vi "CC Rd Wr Observation List.vi"(8 "error in (no error)":errorcluster, 9 "filepath":path, 10 "Write? (F:Read)":bool, 11 "Observation List":T1[](array[typedef])) -> (0 "error out":errorcluster, 1 "file":path, 2 "Errors":string[](array[string]), 3 "Observation List":T1[](array[typedef]))   [LabVIEW 2024]
uses:
  typedefs/CC cluster Observation.ctl
  Observation Queue/CC enum Observation Status.ctl
  Telescope/CC cluster Telescope Offsets.ctl
  typedefs/CC cluster Observation Dither Options.ctl
  typedefs/CC enum Dither Selection.ctl
  typedefs/CC cluster RA and DEC.ctl
  <vilib>/Utility/file.llb/Write Delimited Spreadsheet (string).vi
panel:
  out "Header":string[](array[string])
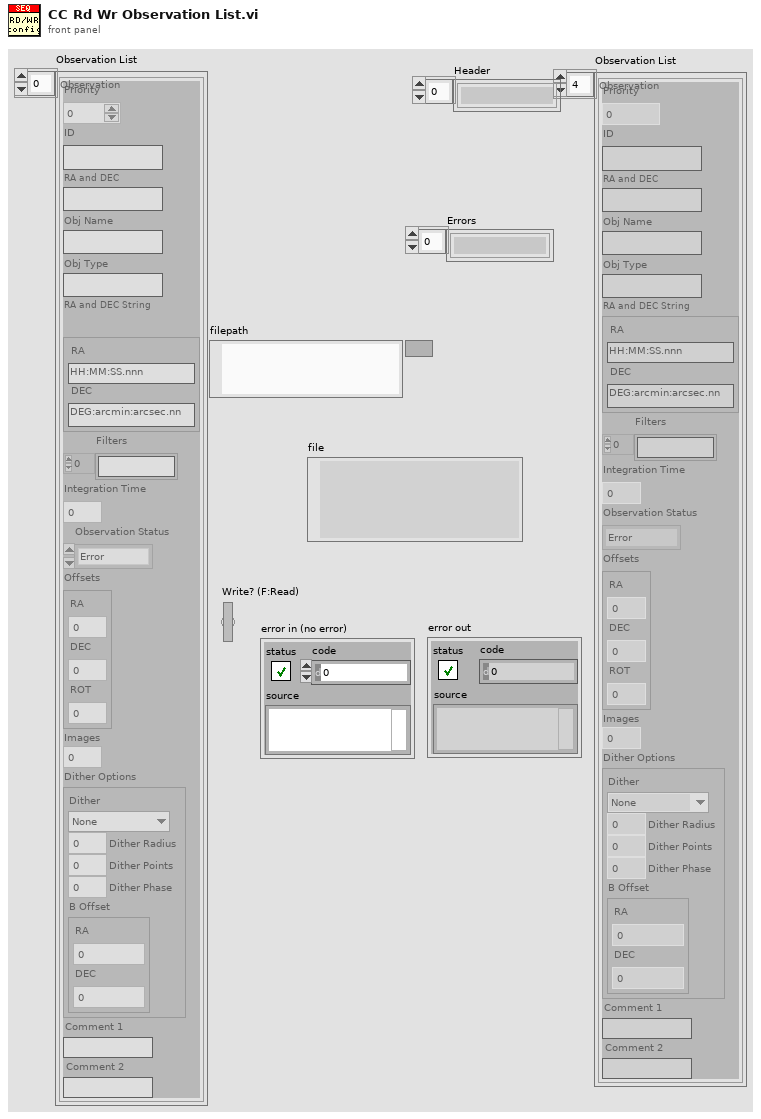
[diagram p1: front panel]
types:
  T1 = typedef "CC cluster Observation.ctl" = cluster{"Priority":i32, "ID":string, "Observer":string, "Obj Name":string, "Obj Type":string, "RA and DEC String":cluster{"RA":string, "DEC":string}, "Filters":string[], "Integration Time":dbl, "Observation Status":T2, "Offsets":T3, "Images":i32, "Dither Options":T4, "Comment 1":string, "Comment 2":string}
  T2 = typedef "CC enum Observation Status.ctl" = enum16{"Ready", "Running", "Done", "Error"}
  T3 = typedef "CC cluster Telescope Offsets.ctl" = cluster{"RA":dbl, "DEC":dbl, "ROT":dbl}
  T4 = typedef "CC cluster Observation Dither Options.ctl" = cluster{"Dither":T5, "Dither Radius":dbl, "Dither Points":i32, "Dither Phase":dbl, "B Offset":T6}
  T5 = typedef "CC enum Dither Selection.ctl" = enum16{"None", "Circle", "Random", "ABBA"}
  T6 = typedef "CC cluster RA and DEC.ctl" = cluster{"RA":dbl, "DEC":dbl}
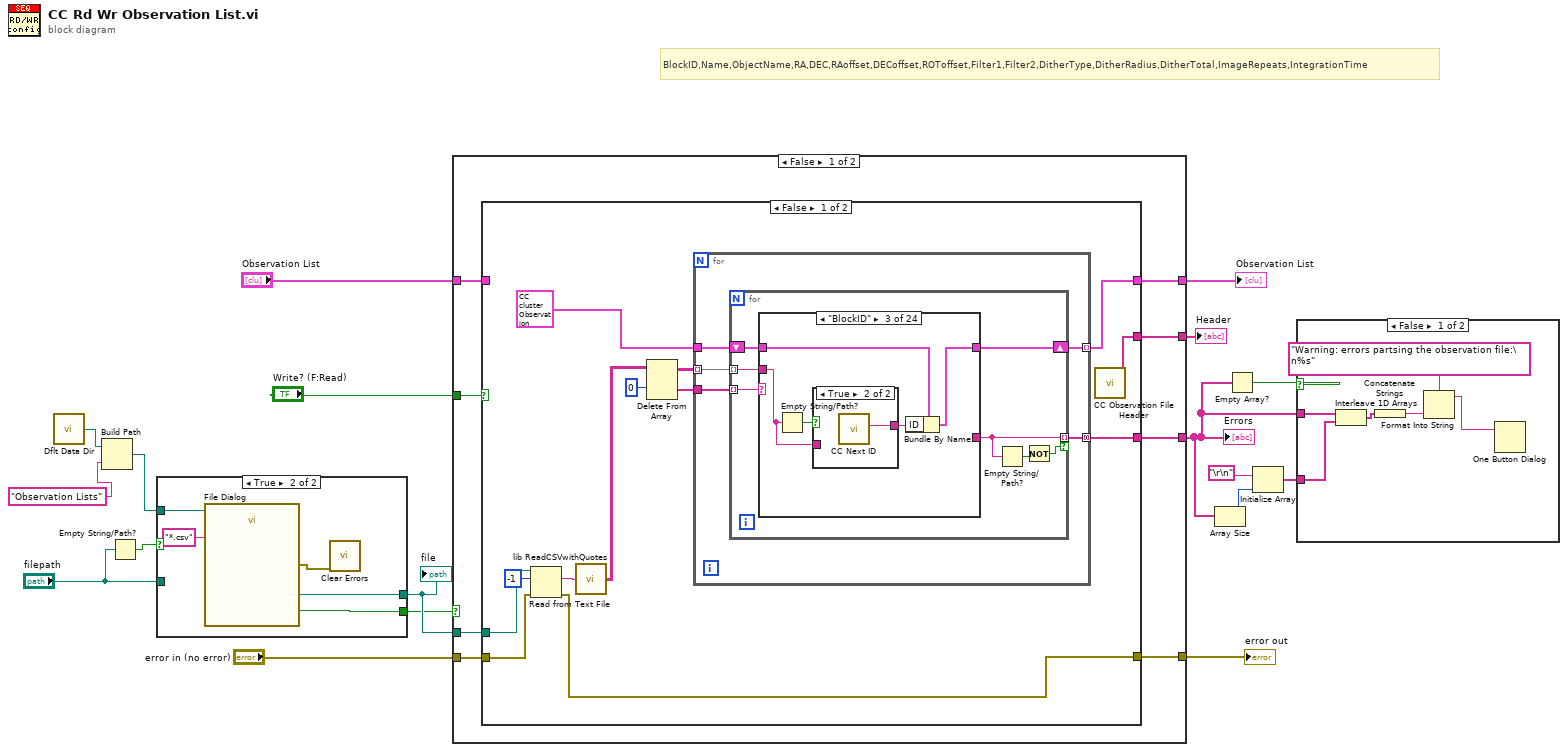
[diagram p0: block diagram]
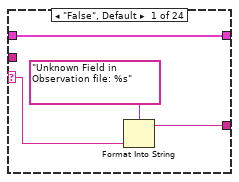
[diagram p3: hidden frame]
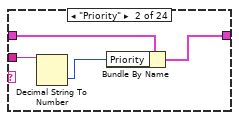
[diagram p4: hidden frame]
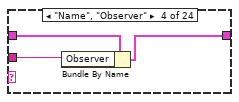
[diagram p6: hidden frame]
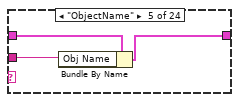
[diagram p7: hidden frame]
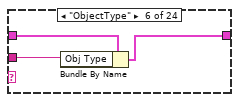
[diagram p8: hidden frame]
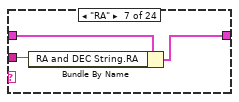
[diagram p9: hidden frame]
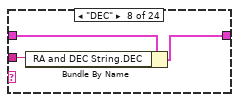
[diagram p10: hidden frame]
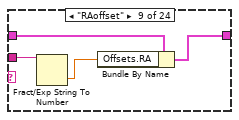
[diagram p11: hidden frame]
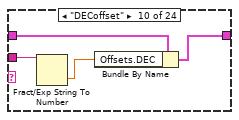
[diagram p12: hidden frame]
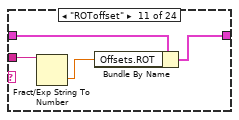
[diagram p13: hidden frame]
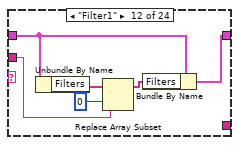
[diagram p14: hidden frame]
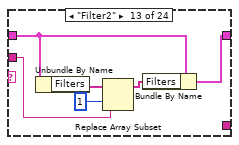
[diagram p15: hidden frame]
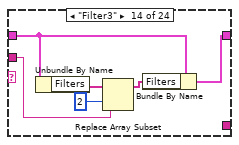
[diagram p16: hidden frame]
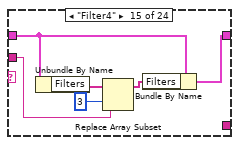
[diagram p17: hidden frame]
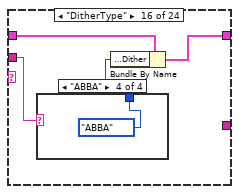
[diagram p18: hidden frame]
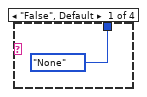
[diagram p19: hidden frame]
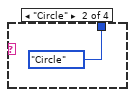
[diagram p20: hidden frame]
diagram:
  # "BlockID,Name,ObjectName,RA,DEC,RAoffset,DECoffset,ROToffset,Filter1,Filter2,DitherType,DitherRadius,DitherTotal,ImageRepeats,IntegrationTime"
  n1 = call <vilib>:"Dflt Data Dir.vi"() -> ("App:Default Data Directory"=w10:path)
  n2 = Build Path(base path=w10, name or relative path="Observation Lists") -> (appended path=w8:path)
  n3 = Empty String/Path?(string/path="filepath") -> (empty?=w13:bool)
  n4 = case shown="True" w13 {
    tunnel: [w19 w24] -> w12
    tunnel: "filepath" -> [w19 _]
    tunnel: w8 -> [_ w23]
    tunnel: [_ w21] -> w7
    frame False {
    }
    frame True {
      n5 = call "File Dialog"("start path"=w23, "pattern (all files)"="*.csv") -> ("selected path"=w24:path, "cancelled"=w21:bool, "error out"=w20:errorcluster)  [unwired: 10 in, 1 out]
      n6 = call <vilib>:"Clear Errors.vi"("error in (no error)"=w20) -> ()  [unwired: 5 in, 2 out]
    }
  }
  "file" <- w12
  n7 = case shown="False" w7 {
    tunnel: "error in (no error)" -> [w32 w193]
    tunnel: "Write? (F:Read)" -> [w31 _]
    tunnel: "Observation List" -> [w30 w194]
    tunnel: [w29 w193] -> w15
    tunnel: [w28 w194] -> w14
    tunnel: w12 -> [w27 _]
    tunnel: [w26 _] -> w3
    tunnel: [w25 _] -> w6
    frame False {
      n8 = case shown="False" w31 {
        tunnel: w32 -> [w33 w192]
        tunnel: w30 -> [_ w188]
        tunnel: w27 -> [w38 w191]
        tunnel: [w34 w190] -> w29
        tunnel: [w41 w188] -> w28
        tunnel: [w40 _] -> w26
        tunnel: [w39 w186] -> w25
        frame False {
          n9 = Read from Text File(file (use dialog)=w38, count=-1, error in=w33) -> (text=w37:string, error out=w34:errorcluster)  [unwired: 1 in, 2 out]
          n10 = call "lib ReadCSVwithQuotes.vi"("String"=w37) -> ("Array"=w35:string[][])  [unwired: 4 in]
          n11 = Delete From Array(array=w35, index (row)=0) -> (deleted portion=w43:string[], array with subset deleted=w42:string[][])  [unwired: 2 in]
          n12 = for {
            tunnel: T1 {"Priority"=0, "ID"="", "Observer"="", "Obj Name"="", "Obj Type"="", "RA and DEC String"={"RA"="12:34:56.789", "DEC"="010:11:12.013"}, "Filters"=["", "", "", ""], "Integration Time"=0.0, "Observation Status"=enum."Ready", "Offsets"={"RA"=0.0, "DEC"=0.0, "ROT"=0.0}, "Images"=0, "Dither Options"={"Dither"=enum."Random", "Dither Radius"=0.0, "Dither Points"=0, "Dither Phase"=0.0, "B Offset"={"RA"=0.0, "DEC"=0.0}}, "Comment 1"="", "Comment 2"=""} ("Observation") -> [w50]
            tunnel: w43 -> [w49]
            tunnel: w42 -> [w48] mode=indexing
            tunnel: [w47] -> w41 mode=indexing
            tunnel: [w46] -> w40 mode=concatenating
            n13 = for {
              shift-right: [w54] -> w47
              shift-left: w50 -> [w55]
              tunnel: w49 -> [w57] mode=indexing
              tunnel: w48 -> [w56] mode=indexing
              tunnel: [w53] -> w46 mode=indexing if=w51
              n14 = case shown="\"BlockID\"" w57 {
                selector: w57 -> [w60 _ _ _ _ _ _ _ _ _ _ _ _ _ _ _ _ _ _ _ _ _ _ _]
                tunnel: w56 -> [_ w63 w66 w73 w76 w79 w82 w85 w89 w93 w97 w100 w106 w112 w118 w125 w133 w139 w154 w168 w172 w176 w180 w183]
                tunnel: w55 -> [w59 w65 w70 w75 w78 w81 w84 w87 w91 w95 w99 w104 w110 w116 w122 w127 w135 w137 w152 w170 w174 w178 w181 w184]
                tunnel: [w59 w64 w69 w74 w77 w80 w83 w86 w90 w94 w98 w105 w111 w117 w123 w126 w134 w140 w155 w169 w173 w177 w179 w182] -> w54
                tunnel: [w58 _ _ _ _ _ _ _ _ _ _ _ _ _ _ _ _ _ _ _ _ _ _ _] -> w53
                frame "False", Default {
                  n15 = Format Into String(format string="Unknown Field in Observation file: %s", w60) -> (resulting string=w58:string)  [unwired: 2 in, 1 out]
                }
                frame "Priority" {
                  n16 = Decimal String To Number(string=w63) -> (number=w62:i32)  [unwired: 2 in, 1 out]
                  n17 = Bundle By Name(cluster=w65, "Priority"=w62) -> (w64:T1)
                }
                frame "BlockID" {
                  n18 = Empty String/Path?(string/path=w66) -> (empty?=w68:bool)
                  n19 = case shown="True" w68 {
                    tunnel: [w71 w72] -> w67
                    tunnel: w66 -> [w71 _]
                    frame False {
                    }
                    frame True {
                      n20 = call "CC Next ID.vi"() -> ("BlockID string"=w72:string)  [unwired: 9 in, 2 out]
                    }
                  }
                  n21 = Bundle By Name(cluster=w70, "ID"=w67) -> (w69:T1)
                }
                frame "Name", "Observer" {
                  n22 = Bundle By Name(cluster=w75, "Observer"=w73) -> (w74:T1)
                }
                frame "ObjectName" {
                  n23 = Bundle By Name(cluster=w78, "Obj Name"=w76) -> (w77:T1)
                }
                frame "ObjectType" {
                  n24 = Bundle By Name(cluster=w81, "Obj Type"=w79) -> (w80:T1)
                }
                frame "RA" {
                  n25 = Bundle By Name(cluster=w84, "RA and DEC String.RA"=w82) -> (w83:T1)
                }
                frame "DEC" {
                  n26 = Bundle By Name(cluster=w87, "RA and DEC String.DEC"=w85) -> (w86:T1)
                }
                frame "RAoffset" {
                  n27 = Fract/Exp String To Number(string=w89) -> (number=w88:dbl)  [unwired: 3 in, 1 out]
                  n28 = Bundle By Name(cluster=w91, "Offsets.RA"=w88) -> (w90:T1)
                }
                frame "DECoffset" {
                  n29 = Fract/Exp String To Number(string=w93) -> (number=w92:dbl)  [unwired: 3 in, 1 out]
                  n30 = Bundle By Name(cluster=w95, "Offsets.DEC"=w92) -> (w94:T1)
                }
                frame "ROToffset" {
                  n31 = Fract/Exp String To Number(string=w97) -> (number=w96:dbl)  [unwired: 3 in, 1 out]
                  n32 = Bundle By Name(cluster=w99, "Offsets.ROT"=w96) -> (w98:T1)
                }
                frame "Filter1" {
                  n33 = Unbundle By Name(w104) -> ("Filters"=w103:string[])
                  n34 = Replace Array Subset(array=w103, new element=w100, index=0) -> (w101:string[])
                  n35 = Bundle By Name(cluster=w104, "Filters"=w101) -> (w105:T1)
                }
                frame "Filter2" {
                  n36 = Unbundle By Name(w110) -> ("Filters"=w109:string[])
                  n37 = Replace Array Subset(array=w109, new element=w106, index=1) -> (w107:string[])
                  n38 = Bundle By Name(cluster=w110, "Filters"=w107) -> (w111:T1)
                }
                frame "Filter3" {
                  n39 = Unbundle By Name(w116) -> ("Filters"=w115:string[])
                  n40 = Replace Array Subset(array=w115, new element=w112, index=2) -> (w113:string[])
                  n41 = Bundle By Name(cluster=w116, "Filters"=w113) -> (w117:T1)
                }
                frame "Filter4" {
                  n42 = Unbundle By Name(w122) -> ("Filters"=w121:string[])
                  n43 = Replace Array Subset(array=w121, new element=w118, index=3) -> (w119:string[])
                  n44 = Bundle By Name(cluster=w122, "Filters"=w119) -> (w123:T1)
                }
                frame "DitherType" {
                  n45 = case shown="\"ABBA\"" w125 {
                    tunnel: [CC_enum_Dither_Selection."None" ("Dither Options.Dither") CC_enum_Dither_Selection."Circle" ("Dither Options.Dither") CC_enum_Dither_Selection."Random" ("Dither Options.Dither") CC_enum_Dither_Selection."ABBA" ("Dither Options.Dither")] -> w124
                    frame "False", Default {
                    }
                    frame "Circle" {
                    }
                    frame "Random" {
                    }
                    frame "ABBA" {
                    }
                  }
                  n46 = Bundle By Name(cluster=w127, "Dither Options.Dither"=w124) -> (w126:T1)
                }
                frame "DitherTotal" {
                  n47 = Decimal String To Number(string=w133) -> (number=w132:i32)  [unwired: 2 in, 1 out]
                  n48 = Bundle By Name(cluster=w135, "Dither Options.Dither Points"=w132) -> (w134:T1)
                }
                frame "DitherX" {
                  n49 = Unbundle By Name(w137) -> ("Dither Options.Dither"=w136:T5)
                  n50 = Fract/Exp String To Number(string=w139) -> (number=w138:dbl)  [unwired: 3 in, 1 out]
                  n51 = case shown="\"Random\"" w136 {
                    tunnel: [w141 w144 w147 w150] -> w140
                    tunnel: w138 -> [_ w143 w146 w149]
                    tunnel: w137 -> [w141 w142 w145 w148]
                    frame "None", Default {
                    }
                    frame "Circle" {
                      n52 = Bundle By Name(cluster=w142, "Dither Options.Dither Radius"=w143) -> (w144:T1)
                    }
                    frame "Random" {
                      n53 = Bundle By Name(cluster=w145, "Dither Options.Dither Radius"=w146) -> (w147:T1)
                    }
                    frame "ABBA" {
                      n54 = Bundle By Name(cluster=w148, "Dither Options.B Offset.RA"=w149) -> (w150:T1)
                    }
                  }
                }
                frame "DitherY" {
                  n55 = Unbundle By Name(w152) -> ("Dither Options.Dither"=w151:T5)
                  n56 = Fract/Exp String To Number(string=w154) -> (number=w153:dbl)  [unwired: 3 in, 1 out]
                  n57 = case shown="\"Random\"" w151 {
                    tunnel: [w156 w159 w162 w166] -> w155
                    tunnel: w153 -> [_ w158 w161 w165]
                    tunnel: w152 -> [w156 w157 w160 w164]
                    frame "None", Default {
                    }
                    frame "Circle" {
                      n58 = Bundle By Name(cluster=w157, "Dither Options.Dither Phase"=w158) -> (w159:T1)
                    }
                    frame "Random" {
                      n59 = Bundle By Name(cluster=w160, "Dither Options.Dither Phase"=w161) -> (w162:T1)
                    }
                    frame "ABBA" {
                      n60 = Bundle By Name(cluster=w164, "Dither Options.B Offset.DEC"=w165, "Dither Options.Dither Points"=4) -> (w166:T1)
                    }
                  }
                }
                frame "DitherPhase" {
                  n61 = Fract/Exp String To Number(string=w168) -> (number=w167:dbl)  [unwired: 3 in, 1 out]
                  n62 = Bundle By Name(cluster=w170, "Dither Options.Dither Phase"=w167) -> (w169:T1)
                }
                frame "Images" {
                  n63 = Decimal String To Number(string=w172) -> (number=w171:i32)  [unwired: 2 in, 1 out]
                  n64 = Bundle By Name(cluster=w174, "Images"=w171) -> (w173:T1)
                }
                frame "IntegrationTime" {
                  n65 = Fract/Exp String To Number(string=w176) -> (number=w175:dbl)  [unwired: 3 in, 1 out]
                  n66 = Bundle By Name(cluster=w178, "Integration Time"=w175) -> (w177:T1)
                }
                frame "Comment1" {
                  n67 = Bundle By Name(cluster=w181, "Comment 1"=w180) -> (w179:T1)
                }
                frame "Comment2" {
                  n68 = Bundle By Name(cluster=w184, "Comment 1"=w183) -> (w182:T1)
                }
              }
              n69 = Empty String/Path?(string/path=w53) -> (empty?=w52:bool)
              n70 = Not(x=w52) -> (.not. x?=w51:bool)
            }
          }
          n71 = call "CC Observation File Header.vi"() -> ("Header"=w39:string[])  [unwired: 10 in, 1 out]
        }
        frame True {
          n72 = call "CC Observation List to Table.vi"("Observation List"=w188) -> ("File Ready Table"=w185:string[][])  [unwired: 7 in, 3 out]
          n73 = call "CC Observation File Header.vi"() -> ("Header"=w186:string[])  [unwired: 10 in, 1 out]
          n74 = Build Array (concatenate)(w186, w185) -> (w187:string[][])
          n75 = call-poly <vilib>:"Write Delimited Spreadsheet.vi"("file path (dialog if empty)"=w191, "2D data"=w187, "error in (no error)"=w192, "delimiter (\\t)"="," ("delimiter (\\t)")) -> ("error out"=w190:errorcluster)  [unwired: 10 in, 1 out]
        }
      }
    }
    frame True {
    }
  }
  "error out" <- w15
  "Observation List" <- w14
  "Errors" <- w3
  "Header" <- w6
  n76 = Array Size(array=w3) -> (size(s)=w2:i32)
  n77 = Empty Array?(array=w3) -> (empty?=w5:bool)
  n78 = Initialize Array("\r\n", w2) -> (w1:string[])
  n79 = case shown="False" w5 {
    tunnel: w3 -> [w200 _]
    tunnel: w1 -> [w199 _]
    frame False {
      n80 = Interleave 1D Arrays(w200, w199) -> (w197:string[])
      n81 = Concatenate Strings(w197) -> (w196:string)
      n82 = Format Into String(format string="Warning: errors partsing the observation file:\n%s", w196) -> (resulting string=w195:string)  [unwired: 2 in, 1 out]
      n83 = One Button Dialog(message=w195) -> ()  [unwired: 1 in, 1 out]
    }
    frame True {
    }
  }
